vi "winForms getChildList.vi"(0 "getParent":bool, 1 "parentType":T1=enum."MSProcess") -> (2 "outputStr":string)   [LabVIEW 2018]
uses:
  winForms parentType.ctl
panel:
  out "parentName":string
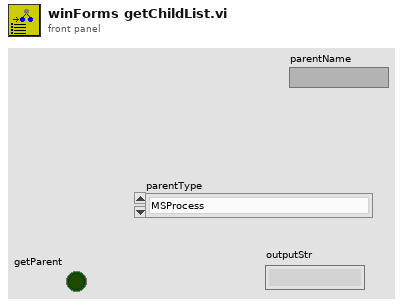
[diagram p1: front panel]
types:
  T1 = typedef "winForms parentType.ctl" = enum16{"none", "MSProcess", "Mathieu", "sp", "gsp", "PriPlt", "SecPlt", "ScanSig", "IonSig", "ionGraph", "mzGraph", "tGraph"}
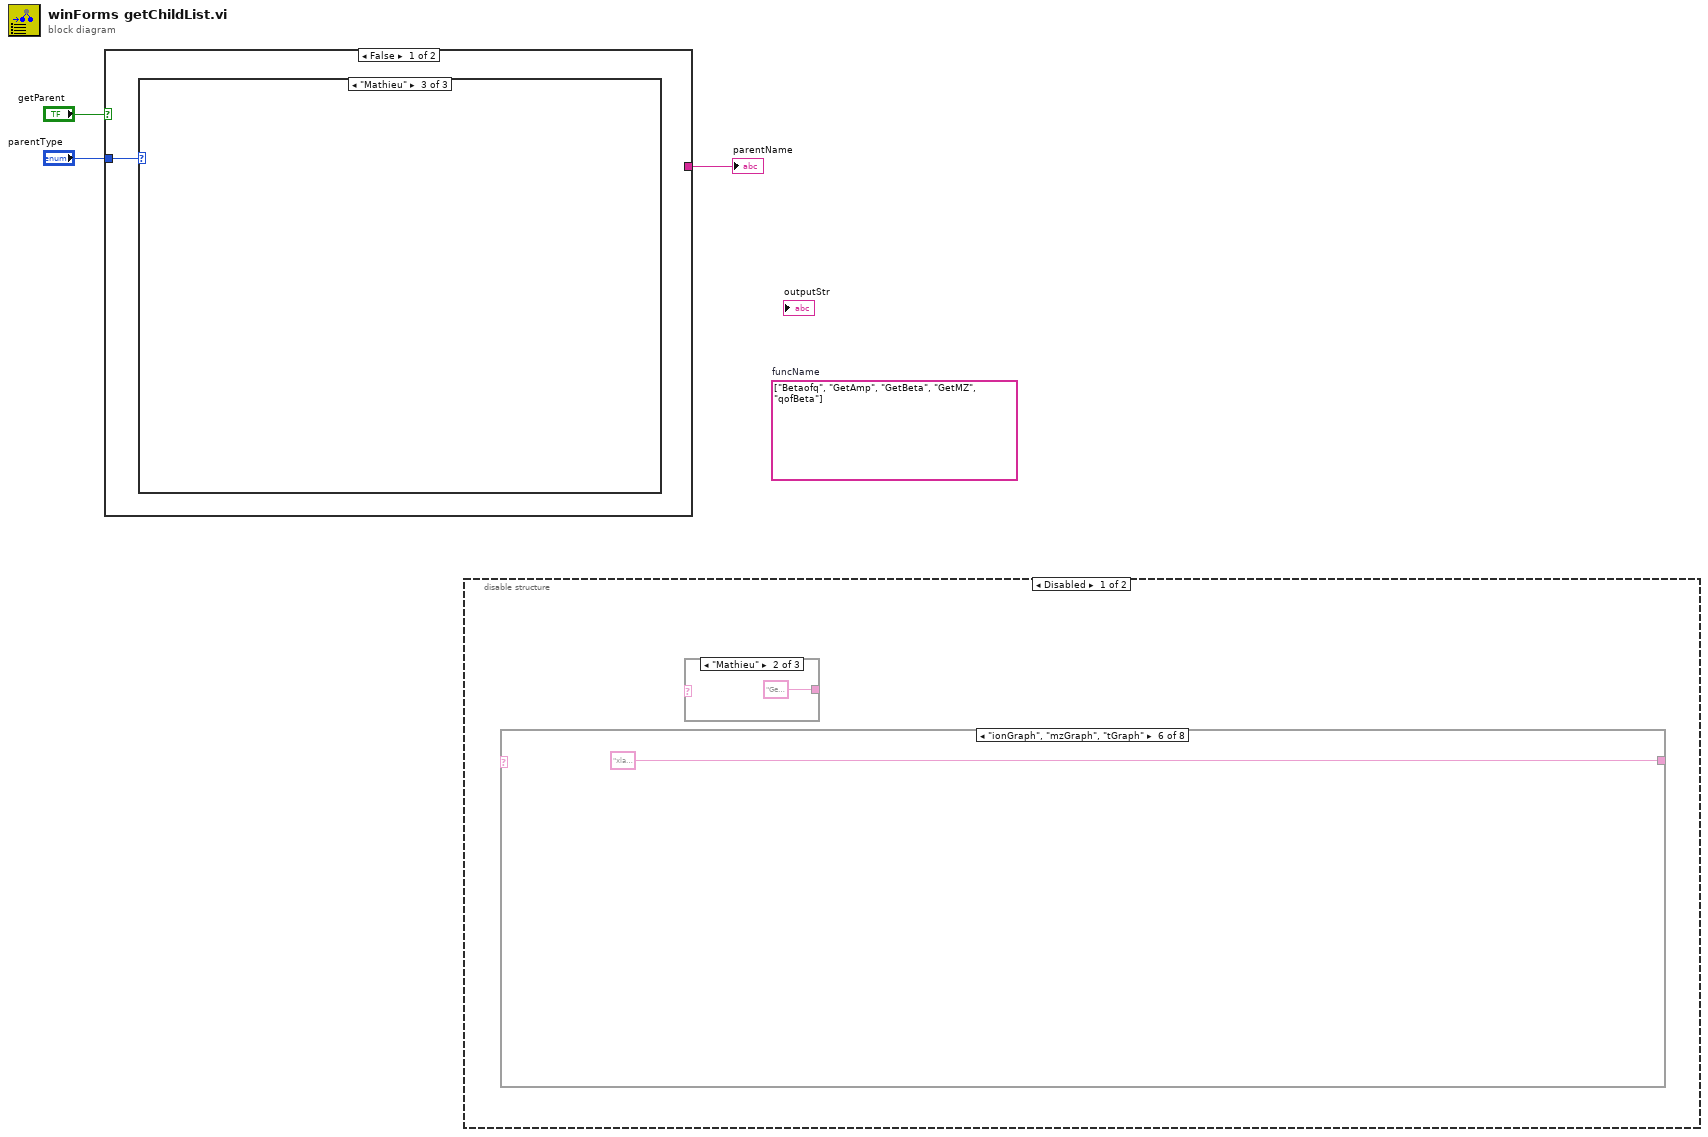
[diagram p0: block diagram]
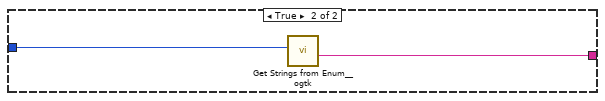
[diagram p4: hidden frame]
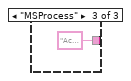
[diagram p6: hidden frame]
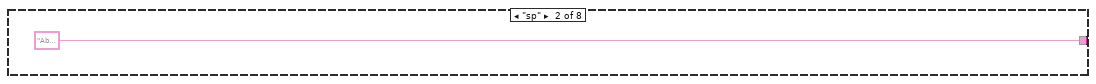
[diagram p8: hidden frame]
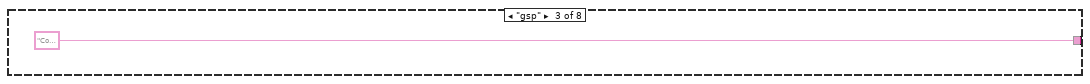
[diagram p9: hidden frame]
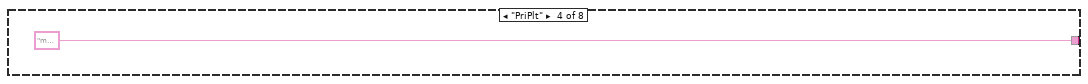
[diagram p10: hidden frame]
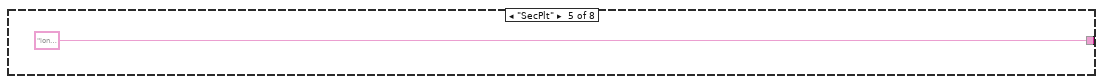
[diagram p11: hidden frame]
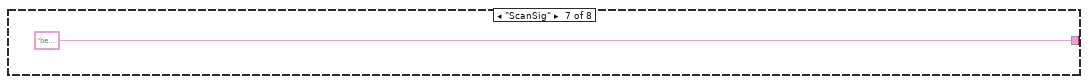
[diagram p12: hidden frame]
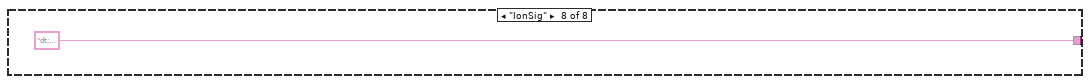
[diagram p13: hidden frame]
diagram:
  (unwired) string[] ["Betaofq", "GetAmp", "GetBeta", "GetMZ", "qofBeta"]  # funcName
  n1 = case shown="False" "getParent" {
    tunnel: "parentType" -> [w4 w6]
    tunnel: [_ w5] -> w2
    frame False {
      n2 = case shown="\"Mathieu\"" w4 {
        frame "none", Default {
        }
        frame "MSProcess" {
        }
        frame "Mathieu" {
        }
      }
    }
    frame True {
      n3 = call <userlib>:"Get Strings from Enum__ogtk.vi"("Enum"=w6) -> ("String Value"=w5:string)  [unwired: 7 in, 3 out]
    }
  }
  "parentName" <- w2
  n4 = disable-structure shown="Disabled" {
    frame Disabled {
      n5 = case shown="\"ionGraph\", \"mzGraph\", \"tGraph\"" {
        selector: _ -> [_ _ _ _ _ _ _ _]
        tunnel: [_ "Abs( signal );Filtering( dt, signal, wintype, winwidth );Negate( signal );NumRectifier( dt, signal );PltAbs( pltSignal );PltFFT( pltSignal );PltFiltering( pltSignal, wintype, winwidth );PltNegate( pltSignal );PltNumRectifier( pltSignal )" "Conv1D( kernel, signal );MakeKernel( dt, kernelType, winWidth );PltConv1D( kernel , pltSignal )" "mzGraph;ScanSig;tGraph" "ionGraph;IonSig" "xlabel;ylabel" "beta;dt;xdata;ydata" "dt;ydata"] -> _
        frame Default {
        }
        frame "sp" {
        }
        frame "gsp" {
        }
        frame "PriPlt" {
        }
        frame "SecPlt" {
        }
        frame "ionGraph", "mzGraph", "tGraph" {
        }
        frame "ScanSig" {
        }
        frame "IonSig" {
        }
      }
      n6 = case shown="\"Mathieu\"" {
        selector: _ -> [_ _ _]
        tunnel: [_ "GetAmp( mz, freq, beta );GetBeta( mz, amp, freq );GetFreq( mz, amp, beta );GetMZ( amp, freq, beta )" "AcqSig( time );AuxScan( auxWfmType, auxStart, iauxCyc, auxCyc, beta, betaScale, auxAmp, auxPulse1, auxPulse2, auxPulseAmp, time );CLFreqScan( targetfreq, time );FGen( amp, freq );Header( ionTrapR0, ionTrapZ0, priRFMaxAmp );IonGate( trialTime, TPH, enableAGC );LaserTrig( trigFreq, phaseDeg, shots );LinearAmpScan( auxWfmType, iauxCyc, beta, betaScale, auxAmp, auxPulse1, auxPulse2, auxPulseAmp, time, amp, continuous );PhaseScan( auxWfmType, auxStart, iauxCyc, auxCyc, beta, betaScale, auxAmp, auxPulse1, auxPulse2, auxPulseAmp, time, freq, stepWidth );PhaseScanII( auxWfmType, auxStart, iauxCyc, auxCyc, beta, betaScale, auxAmp, auxPulse1, auxPulse2, auxPulseAmp, dm, freq, stepWidth );ResetRFPhase( iniPhase );RFStart( freq, amp, wfmType );RFStop();SetDAQ( channel, sampRate );UpdAO( func, val );UpdAuxArbPulses( cycleIni, cycleEnd, pulseInt );UpdConj( iniPhase, conjLen, phaseDiff, fixedLen );UpdDO( func, val );UpdIGVolts( onVolt, offVolt );UpdRFChBias( ch1, ch2, ch3 );UpdRFChFunc( ch1, ch2, ch3 );UpdRFChScale( ch1, ch2, ch3 );Wait( timeout, DI, edge )"] -> _
        frame Default {
        }
        frame "Mathieu" {
        }
        frame "MSProcess" {
        }
      }
    }
    frame Enabled {
    }
  }
